vi "globalTearDown.vi"(8 "error in":errorcluster, 11 "Loopback in":refnum<class "Loopback.lvclass">) -> (0 "error out":errorcluster, 3 "Loopback out":refnum<class "Loopback.lvclass">)   [LabVIEW 2020, in "Loopback.lvclass"]
uses:
  Loopback.lvclass
  Loopback.lvclass/Loopback.ctl
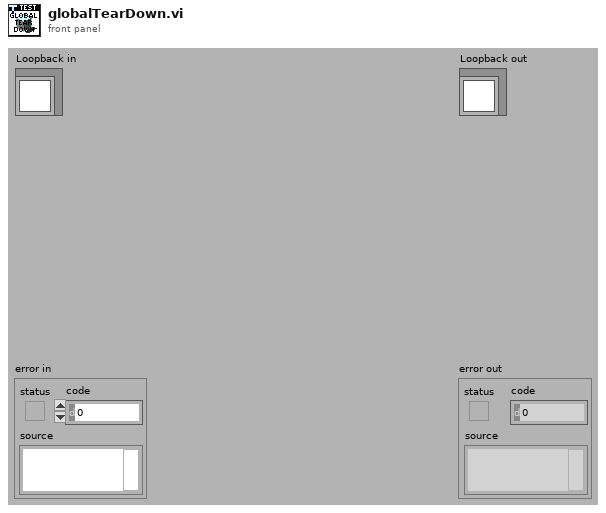
[diagram p1: front panel]
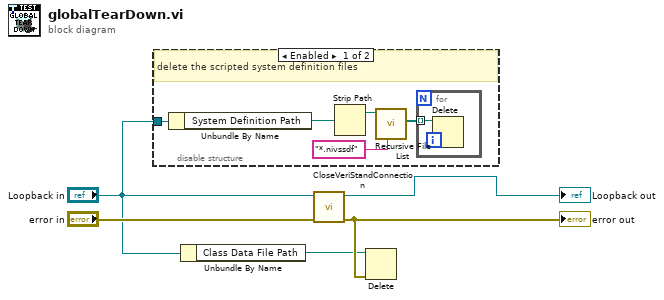
[diagram p0: block diagram]
diagram:
  n1 = disable-structure shown="Enabled" {
    disable-tunnel: "Loopback in" -> [w10 _]
    frame Enabled {
      # "delete the scripted system definition files"
      n2 = Unbundle By Name(w10) -> ("System Definition Path"=w7:path)
      n3 = Strip Path(path=w7) -> (stripped path=w6:path)  [unwired: 1 out]
      n4 = call <vilib>:"Recursive File List.vi"("pattern"="*.nivssdf", "Folder Path"=w6) -> ("All Files in Dir"=w8:path[])  [unwired: 5 in, 4 out]
      n5 = for {
        tunnel: w8 -> [w11] mode=indexing
        n6 = Delete(path (use dialog)=w11) -> ()  [unwired: 4 in, 3 out]
      }
    }
    frame Disabled {
    }
  }
  n7 = Unbundle By Name("Loopback in") -> ("Class Data File Path"=w1:path)
  n8 = call-dynamic "CloseVeriStandConnection.vi"("error in (no error)"="error in", "VeriStand Test Case in"="Loopback in") -> ("error out"=w3:errorcluster, "VeriStand Test Case out"=→"Loopback out":refnum<class "Loopback.lvclass">)  [unwired: 8 in]
  "error out" <- w3
  n9 = Delete(path (use dialog)=w1, error in=w3) -> ()  [unwired: 3 in, 3 out]
